vi "Core1.vi"(8 "error in (no error)":errorcluster, 11 "MB in":refnum<class "WebSocket Client CR.lvclass">) -> (0 "consumer error":errorcluster, 3 "MB out":refnum<class "WebSocket Client CR.lvclass">)   [LabVIEW 2021, in "WebSockets.lvlib" / "WebSocket Client CR.lvclass"]
uses:
  WebSocket Client CR.lvclass
  WebSocket Client CR.lvclass/WebSocket Client CR.ctl
  ctl/CR_Core_State.ctl
panel:
  out "MHL error":errorcluster
  in  "write enable":bool=TRUE
  out "CR_Core_State":T1=enum."requests"
  in  "stop":bool
  out "stopped":bool
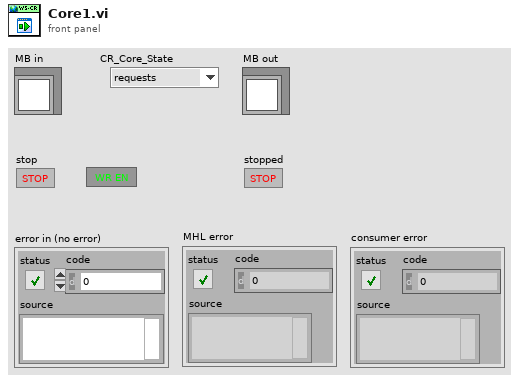
[diagram p1: front panel]
types:
  T1 = typedef "WebSockets.lvlib/WebSocket Client CR.lvclass/CR_Core_State.ctl" = enum8{"initialization", "redefine", "standby", "ping", "connect", "wait to reconnect", "wait to reset timeout", "configure", "requests", "close connection", "stop"}
  T2 = typedef "WebSockets.lvlib/WebSocket Client CR.lvclass/MB timeouts.ctl" = cluster{"reconn_timeout":i32, "N attempt max":i32, "t_reset_TTL":i32, "period":i32}
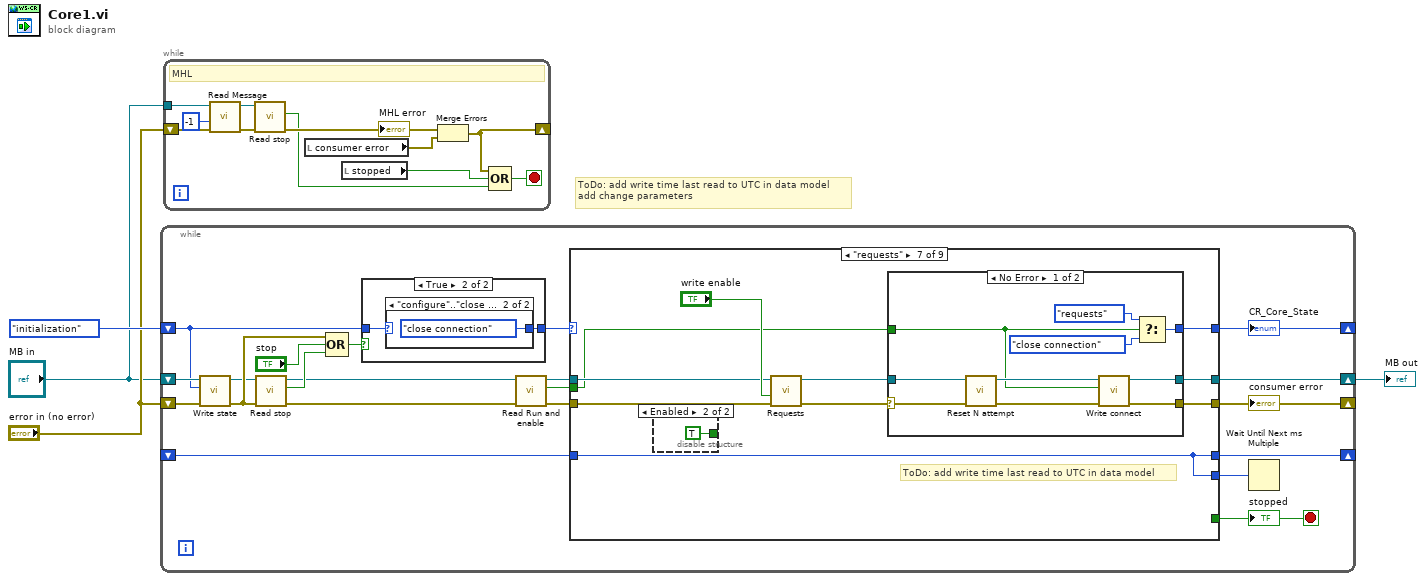
[diagram p0: block diagram]
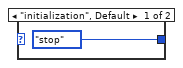
[diagram p3: hidden frame]
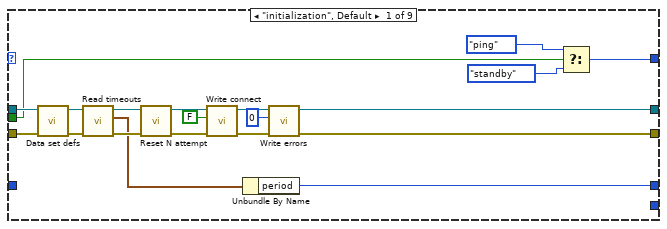
[diagram p4: hidden frame]
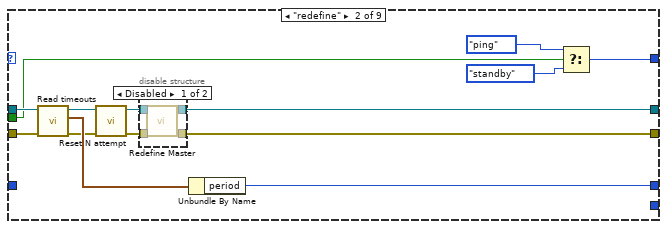
[diagram p5: hidden frame]
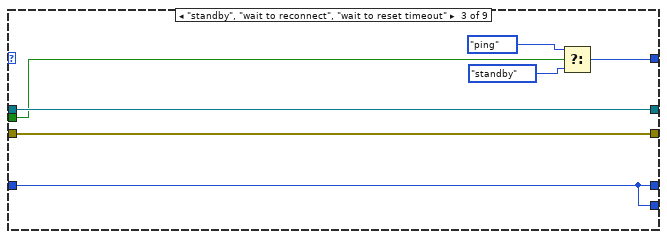
[diagram p7: hidden frame]
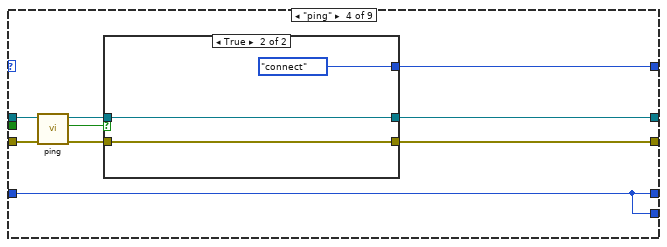
[diagram p8: hidden frame]
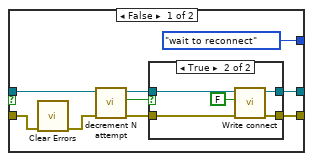
[diagram p9: hidden frame]
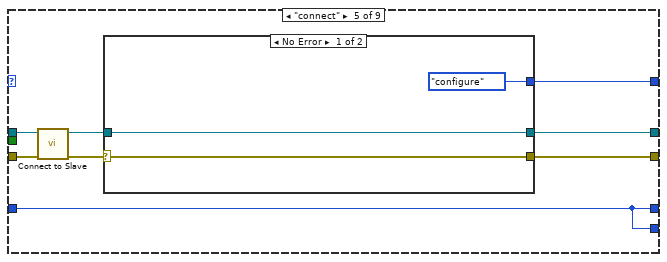
[diagram p11: hidden frame]
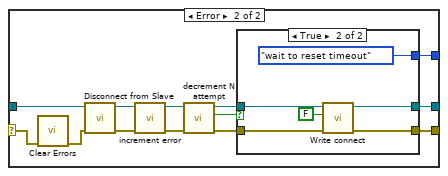
[diagram p12: hidden frame]
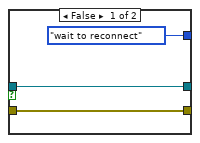
[diagram p13: hidden frame]
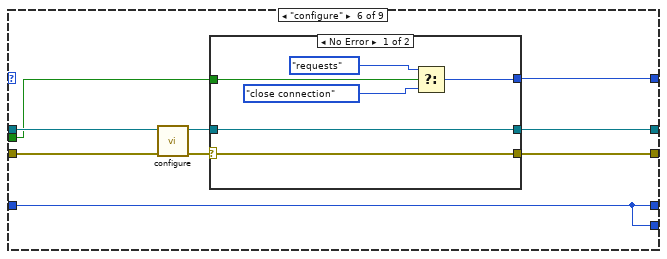
[diagram p14: hidden frame]
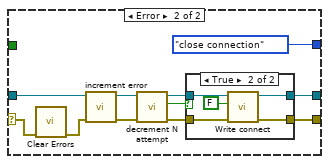
[diagram p15: hidden frame]
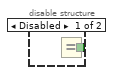
[diagram p17: hidden frame]
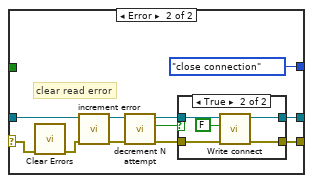
[diagram p18: hidden frame]
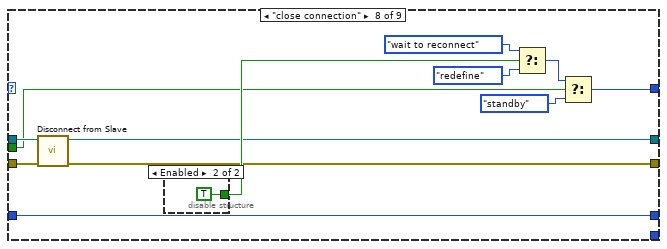
[diagram p20: hidden frame]
diagram:
  # "ToDo: add write time last read to UTC in data model\nadd change parameters"
  n1 = while {
    shift-right: [w22] -> w4
    shift-left: "MB in" -> [w15]
    shift-right: [w20] -> _
    shift-left: "error in (no error)" -> [w14]
    shift-right: [w24] -> _
    shift-left: _ -> [w25]
    shift-right: [w21] -> _
    shift-left: CR_Core_State."initialization" ("state") -> [w6]
    stop <- w19 stop-if-true
    n2 = call "Write state.vi"("error in (no error)"=w14, "state"=w6, "Master CR in"=w15) -> ("error out"=w10:errorcluster, "Master CR out"=w9:refnum<class "WebSocket Client CR.lvclass">)  [unwired: 7 in]
    n3 = call "Read stop.vi"("error in (no error)"=w10, "Master CR in"=w9) -> ("error out"=w7:errorcluster, "Stop"=w12:bool, "Master CR out"=w8:refnum<class "WebSocket Client CR.lvclass">)  [unwired: 7 in]
    n4 = Compound Arithmetic op=OR(w10, "stop", w12) -> (w11:bool)
    n5 = case shown="True" w11 {
      tunnel: w6 -> [w26 w28]
      tunnel: [w26 w27] -> w5
      frame False {
      }
      frame True {
        n6 = case shown="\"configure\"..\"close connection\"" w28 {
          tunnel: [CR_Core_State."stop" ("MB_TCP_State") CR_Core_State."close connection" ("MB_TCP_State")] -> w27
          frame "initialization", Default {
          }
          frame "configure".."close connection" {
          }
        }
      }
    }
    n7 = call "Read Run and enable.vi"("error in (no error)"=w7, "Master CR in"=w8) -> ("error out"=w18:errorcluster, "Enable and Run"=w16:bool, "Master CR out"=w17:refnum<class "WebSocket Client CR.lvclass">)  [unwired: 7 in]
    n8 = case shown="\"requests\"" w5 {
      tunnel: [_ _ _ _ _ _ _ _ TRUE] -> w19
      tunnel: w17 -> [w48 w61 w74 w82 w109 w141 w174 w222 w229]
      tunnel: [w33 w53 w74 w86 w113 w147 w181 w214 w232] -> w22
      tunnel: w18 -> [w49 w60 w73 w81 w110 w140 w173 w221 w228]
      tunnel: [w34 w62 w75 w85 w112 w146 w180 w215 CR_Core_State."initialization" ("MB_TCP_State")] -> w21
      tunnel: [w32 w52 w73 w84 w111 w145 w179 w213 w231] -> w20
      tunnel: [w50 w58 w71 w83 w106 w144 w177 w223 w236] -> w24
      tunnel: w25 -> [_ _ w71 w83 w106 w144 w177 w223 w236]
      tunnel: [_ _ w71 w83 w106 w144 w177 _ _] -> w23
      tunnel: w16 -> [w31 w51 w72 _ _ w139 w172 w212 _]
      frame "initialization", Default {
        n9 = call "Data set defs.vi"("error in (no error)"=w49, "Master CR in"=w48) -> ("error out"=w43:errorcluster, "Master CR out"=w46:refnum<class "WebSocket Client CR.lvclass">)  [unwired: 8 in]
        n10 = call "Read timeouts.vi"("error in (no error)"=w43, "Master CR in"=w46) -> ("error out"=w47:errorcluster, "MB timeouts"=w44:T2, "Master CR out"=w45:refnum<class "WebSocket Client CR.lvclass">)  [unwired: 7 in]
        n11 = call "Reset N attempt.vi"("error in (no error)"=w47, "Master CR in"=w45) -> ("error out"=w41:errorcluster, "Master CR out"=w42:refnum<class "WebSocket Client CR.lvclass">)  [unwired: 8 in]
        n12 = call "Write connect.vi"("error in (no error)"=w41, "connect"=FALSE, "Master CR in"=w42) -> ("error out"=w39:errorcluster, "Master CR out"=w38:refnum<class "WebSocket Client CR.lvclass">)  [unwired: 7 in]
        n13 = Unbundle By Name(w44) -> ("period"=w50:i32)
        n14 = call "Write errors.vi"("error in (no error)"=w39, "errors"=0, "Master CR in"=w38) -> ("error out"=w32:errorcluster, "Master CR out"=w33:refnum<class "WebSocket Client CR.lvclass">)  [unwired: 7 in]
        n15 = Select(t=CR_Core_State."ping" ("MB_TCP_State"), s=w31, f=CR_Core_State."standby" ("MB_TCP_State")) -> (s? t:f=w34:T1)
      }
      frame "redefine" {
        n16 = call "Read timeouts.vi"("error in (no error)"=w60, "Master CR in"=w61) -> ("error out"=w57:errorcluster, "MB timeouts"=w59:T2, "Master CR out"=w56:refnum<class "WebSocket Client CR.lvclass">)  [unwired: 7 in]
        n17 = call "Reset N attempt.vi"("error in (no error)"=w57, "Master CR in"=w56) -> ("error out"=w54:errorcluster, "Master CR out"=w55:refnum<class "WebSocket Client CR.lvclass">)  [unwired: 8 in]
        n18 = disable-structure shown="Disabled" {
          disable-tunnel: w55 -> [w68 w70]
          disable-tunnel: w54 -> [w67 w69]
          disable-tunnel: [w66 w70] -> w53
          disable-tunnel: [w65 w69] -> w52
          frame Disabled {
            n19 = call "Redefine Master.vi"("error in (no error)"=w67, "Master CR in"=w68) -> ("error out"=w65:errorcluster, "Master CR out"=w66:refnum<class "WebSocket Client CR.lvclass">)  [unwired: 8 in]
          }
          frame Enabled {
          }
        }
        n20 = Unbundle By Name(w59) -> ("period"=w58:i32)
        n21 = Select(t=CR_Core_State."ping" ("MB_TCP_State"), s=w51, f=CR_Core_State."standby" ("MB_TCP_State")) -> (s? t:f=w62:T1)
      }
      frame "standby", "wait to reconnect", "wait to reset timeout" {
        n22 = Select(t=CR_Core_State."ping" ("MB_TCP_State"), s=w72, f=CR_Core_State."standby" ("MB_TCP_State")) -> (s? t:f=w75:T1)
      }
      frame "ping" {
        n23 = call-dynamic "ping.vi"("error in (no error)"=w81, "MB_TCP in"=w82) -> ("error out"=w78:errorcluster, "Ping OK"=w79:bool, "MB_TCP out"=w80:refnum<class "WebSocket Client CR.lvclass">)  [unwired: 7 in]
        n24 = case shown="True" w79 {
          tunnel: w80 -> [w89 w105]
          tunnel: [CR_Core_State."wait to reconnect" ("MB_TCP_State") CR_Core_State."connect" ("MB_TCP_State")] -> w85
          tunnel: [w94 w105] -> w86
          tunnel: [w93 w103] -> w84
          tunnel: w78 -> [w90 w103]
          frame False {
            n25 = call <vilib>:"Clear Errors.vi"("error in (no error)"=w90) -> ("error out"=w88:errorcluster)  [unwired: 5 in, 1 out]
            n26 = call "decrement N attempt.vi"("error in (no error)"=w88, "Master CR in"=w89) -> ("error out"=w91:errorcluster, "=0"=w95:bool, "Master CR out"=w92:refnum<class "WebSocket Client CR.lvclass">)  [unwired: 7 in]
            n27 = case shown="True" w95 {
              tunnel: w92 -> [w97 w99]
              tunnel: [w97 w102] -> w94
              tunnel: w91 -> [w96 w98]
              tunnel: [w96 w100] -> w93
              frame False {
              }
              frame True {
                n28 = call "Write connect.vi"("error in (no error)"=w98, "connect"=FALSE, "Master CR in"=w99) -> ("error out"=w100:errorcluster, "Master CR out"=w102:refnum<class "WebSocket Client CR.lvclass">)  [unwired: 7 in]
              }
            }
          }
          frame True {
          }
        }
      }
      frame "connect" {
        n29 = call-dynamic "Connect to Slave.vi"("error in (no error)"=w110, "network master in"=w109) -> ("error out"=w107:errorcluster, "network master out"=w108:refnum<class "WebSocket Client CR.lvclass">)  [unwired: 8 in]
        n30 = case shown="No Error" w107 {
          selector: w107 -> [w114 w121]
          tunnel: w108 -> [w115 w122]
          tunnel: [CR_Core_State."configure" ("MB_TCP_State") w127] -> w112
          tunnel: [w115 w126] -> w113
          tunnel: [w114 w125] -> w111
          frame No Error {
          }
          frame Error {
            n31 = call <vilib>:"Clear Errors.vi"("error in (no error)"=w121) -> ("error out"=w120:errorcluster)  [unwired: 5 in, 1 out]
            n32 = call-dynamic "Disconnect from Slave.vi"("error in (no error)"=w120, "network master in"=w122) -> ("error out"=w123:errorcluster, "network master out"=w124:refnum<class "WebSocket Client CR.lvclass">)  [unwired: 8 in]
            n33 = call "increment error.vi"("error in (no error)"=w123, "Master CR in"=w124) -> ("error out"=w119:errorcluster, "Master CR out"=w129:refnum<class "WebSocket Client CR.lvclass">)  [unwired: 7 in, 1 out]
            n34 = call "decrement N attempt.vi"("error in (no error)"=w119, "Master CR in"=w129) -> ("error out"=w117:errorcluster, "=0"=w128:bool, "Master CR out"=w118:refnum<class "WebSocket Client CR.lvclass">)  [unwired: 7 in]
            n35 = case shown="True" w128 {
              tunnel: [CR_Core_State."wait to reconnect" ("MB_TCP_State") CR_Core_State."wait to reset timeout" ("MB_TCP_State")] -> w127
              tunnel: w118 -> [w131 w134]
              tunnel: [w131 w137] -> w126
              tunnel: w117 -> [w130 w133]
              tunnel: [w130 w135] -> w125
              frame False {
              }
              frame True {
                n36 = call "Write connect.vi"("error in (no error)"=w133, "connect"=FALSE, "Master CR in"=w134) -> ("error out"=w135:errorcluster, "Master CR out"=w137:refnum<class "WebSocket Client CR.lvclass">)  [unwired: 7 in]
              }
            }
          }
        }
      }
      frame "configure" {
        n37 = call-dynamic "configure.vi"("error in (no error)"=w140, "Master CR in"=w141) -> ("error out"=w142:errorcluster, "Master CR out"=w143:refnum<class "WebSocket Client CR.lvclass">)  [unwired: 8 in]
        n38 = case shown="No Error" w142 {
          selector: w142 -> [w148 w163]
          tunnel: [w153 CR_Core_State."close connection" ("MB_TCP_State")] -> w146
          tunnel: [w148 w156] -> w145
          tunnel: w143 -> [w149 w155]
          tunnel: [w149 w157] -> w147
          tunnel: w139 -> [w150 _]
          frame No Error {
            n39 = Select(t=CR_Core_State."requests" ("MB_TCP_State"), s=w150, f=CR_Core_State."close connection" ("MB_TCP_State")) -> (s? t:f=w153:T1)
          }
          frame Error {
            n40 = call <vilib>:"Clear Errors.vi"("error in (no error)"=w163) -> ("error out"=w154:errorcluster)  [unwired: 5 in, 1 out]
            n41 = call "increment error.vi"("error in (no error)"=w154, "Master CR in"=w155) -> ("error out"=w159:errorcluster, "Master CR out"=w158:refnum<class "WebSocket Client CR.lvclass">)  [unwired: 7 in, 1 out]
            n42 = call "decrement N attempt.vi"("error in (no error)"=w159, "Master CR in"=w158) -> ("error out"=w160:errorcluster, "=0"=w162:bool, "Master CR out"=w161:refnum<class "WebSocket Client CR.lvclass">)  [unwired: 7 in]
            n43 = case shown="True" w162 {
              tunnel: w161 -> [w166 w171]
              tunnel: [w166 w170] -> w157
              tunnel: w160 -> [w165 w169]
              tunnel: [w165 w167] -> w156
              frame False {
              }
              frame True {
                n44 = call "Write connect.vi"("error in (no error)"=w169, "connect"=FALSE, "Master CR in"=w171) -> ("error out"=w167:errorcluster, "Master CR out"=w170:refnum<class "WebSocket Client CR.lvclass">)  [unwired: 7 in]
              }
            }
          }
        }
      }
      frame "requests" {
        # "ToDo: add write time last read to UTC in data model"
        n45 = disable-structure shown="Enabled" {
          disable-tunnel: [w182 TRUE] -> _
          frame Disabled {
            n46 = Equal?() -> (x = y?=w182:bool)  [unwired: 2 in]
          }
          frame Enabled {
          }
        }
        n47 = call-dynamic "Requests.vi"("error in (no error)"=w173, "write enable"="write enable", "TCP Client in"=w174) -> ("error out"=w176:errorcluster, "MB_TCP out"=w178:refnum<class "WebSocket Client CR.lvclass">)  [unwired: 7 in]
        n48 = case shown="No Error" w176 {
          selector: w176 -> [w189 w204]
          tunnel: [w193 CR_Core_State."close connection" ("MB_TCP_State")] -> w180
          tunnel: w172 -> [w186 _]
          tunnel: [w184 w200] -> w179
          tunnel: w178 -> [w190 w197]
          tunnel: [w187 w201] -> w181
          frame No Error {
            n49 = call "Reset N attempt.vi"("error in (no error)"=w189, "Master CR in"=w190) -> ("error out"=w185:errorcluster, "Master CR out"=w188:refnum<class "WebSocket Client CR.lvclass">)  [unwired: 8 in]
            n50 = call "Write connect.vi"("error in (no error)"=w185, "connect"=w186, "Master CR in"=w188) -> ("error out"=w184:errorcluster, "Master CR out"=w187:refnum<class "WebSocket Client CR.lvclass">)  [unwired: 7 in]
            n51 = Select(t=CR_Core_State."requests" ("MB_TCP_State"), s=w186, f=CR_Core_State."close connection" ("MB_TCP_State")) -> (s? t:f=w193:T1)
          }
          frame Error {
            # "clear read error"
            n52 = call <vilib>:"Clear Errors.vi"("error in (no error)"=w204) -> ("error out"=w196:errorcluster)  [unwired: 5 in, 1 out]
            n53 = call "increment error.vi"("error in (no error)"=w196, "Master CR in"=w197) -> ("error out"=w198:errorcluster, "Master CR out"=w203:refnum<class "WebSocket Client CR.lvclass">)  [unwired: 7 in, 1 out]
            n54 = call "decrement N attempt.vi"("error in (no error)"=w198, "Master CR in"=w203) -> ("error out"=w199:errorcluster, "=0"=w195:bool, "Master CR out"=w202:refnum<class "WebSocket Client CR.lvclass">)  [unwired: 7 in]
            n55 = case shown="True" w195 {
              tunnel: w202 -> [w206 w211]
              tunnel: [w206 w210] -> w201
              tunnel: w199 -> [w205 w209]
              tunnel: [w205 w207] -> w200
              frame False {
              }
              frame True {
                n56 = call "Write connect.vi"("error in (no error)"=w209, "connect"=FALSE, "Master CR in"=w211) -> ("error out"=w207:errorcluster, "Master CR out"=w210:refnum<class "WebSocket Client CR.lvclass">)  [unwired: 7 in]
              }
            }
          }
        }
      }
      frame "close connection" {
        n57 = call-dynamic "Disconnect from Slave.vi"("error in (no error)"=w221, "network master in"=w222) -> ("error out"=w213:errorcluster, "network master out"=w214:refnum<class "WebSocket Client CR.lvclass">)  [unwired: 8 in]
        n58 = disable-structure shown="Enabled" {
          disable-tunnel: [w224 TRUE] -> w216
          frame Disabled {
            n59 = Equal?() -> (x = y?=w224:bool)  [unwired: 2 in]
          }
          frame Enabled {
          }
        }
        n60 = Select(t=CR_Core_State."wait to reconnect" ("MB_TCP_State"), s=w216, f=CR_Core_State."redefine" ("MB_TCP_State")) -> (s? t:f=w218:T1)
        n61 = Select(t=w218, s=w212, f=CR_Core_State."standby" ("MB_TCP_State")) -> (s? t:f=w215:T1)
      }
      frame "stop" {
        n62 = call "Write connect.vi"("error in (no error)"=w228, "connect"=FALSE, "Master CR in"=w229) -> ("error out"=w227:errorcluster, "Master CR out"=w226:refnum<class "WebSocket Client CR.lvclass">)  [unwired: 7 in]
        n63 = call "Write stop.vi"("error in (no error)"=w227, "Stop"=FALSE, "Master CR in"=w226) -> ("error out"=w231:errorcluster, "Master CR out"=w232:refnum<class "WebSocket Client CR.lvclass">)  [unwired: 7 in]
      }
    }
    "CR_Core_State" <- w21
    "consumer error" <- w20
    "stopped" <- w19
    n64 = Wait Until Next ms Multiple(millisecond multiple=w23) -> ()  [unwired: 1 out]
  }
  "MB out" <- w4
  n65 = while {
    tunnel: "MB in" -> [w245]
    shift-right: [w240] -> _
    shift-left: "error in (no error)" -> [w244]
    stop <- w238 stop-if-true
    # "MHL"
    n66 = call "Read Message.vi"("error in (no error)"=w244, "timeout (0)"=-1, "Master CR in"=w245) -> ("error out"=w243:errorcluster, "Master CR out"=w242:refnum<class "WebSocket Client CR.lvclass">)  [unwired: 6 in, 1 out]
    n67 = call "Read stop.vi"("error in (no error)"=w243, "Master CR in"=w242) -> ("error out"=w241:errorcluster, "Stop"=w239:bool)  [unwired: 7 in, 1 out]
    "MHL error" <- w241
    n68 = local read "consumer error"() -> (w246:errorcluster)
    n69 = local read "stopped"() -> (w237:bool)
    n70 = Merge Errors(w241, w246) -> (w240:errorcluster)
    n71 = Compound Arithmetic op=OR(w240, w237, w239) -> (w238:bool)
  }
